vi "create_roi_file.vi"(7 "Data Files Path":path=path "C:/Users/QCC/Documents/Cesium_project/LabVIEW Projects/data/2011_03_02", 8 "error in (no error)":errorcluster, 9 "iteration string":string, 10 "date/time string":string, 11 "Camera in":refnum<class "Camera.lvclass">) -> (0 "error out":errorcluster, 3 "Camera out":refnum<class "Camera.lvclass">)   [LabVIEW 2013, in "Camera.lvclass"]
uses:
  Camera.lvclass
  Camera.lvclass/Camera.ctl
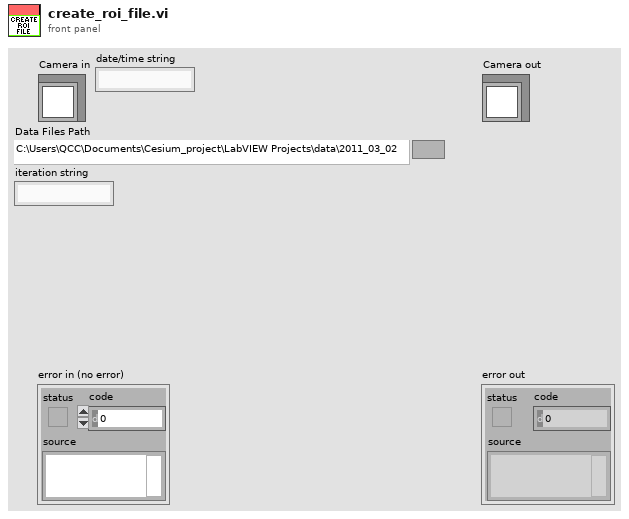
[diagram p1: front panel]
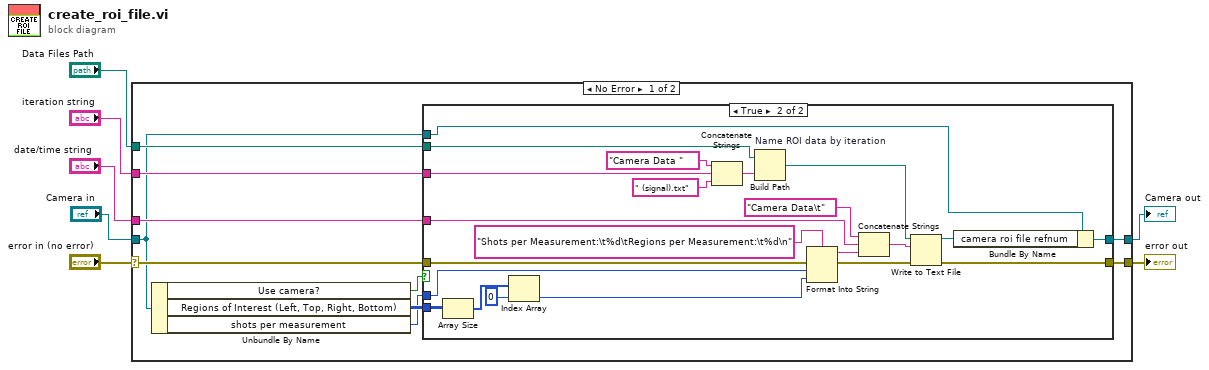
[diagram p0: block diagram]
diagram:
  n1 = case shown="No Error" "error in (no error)" {
    selector: "error in (no error)" -> [w15 w43]
    tunnel: [w14 w43] -> w6
    tunnel: [w8 w42] -> w4
    tunnel: "Camera in" -> [w9 w42]
    tunnel: "Data Files Path" -> [w17 _]
    tunnel: "date/time string" -> [w16 _]
    tunnel: "iteration string" -> [w13 _]
    frame No Error {
      n2 = Unbundle By Name(w9) -> ("Use camera?"=w12:bool, "Regions of Interest (Left, Top, Right, Bottom)"=w11:i32[][], "shots per measurement"=w10:i32)
      n3 = case shown="True" w12 {
        tunnel: w17 -> [_ w32]
        tunnel: w16 -> [_ w31]
        tunnel: w15 -> [w19 w28]
        tunnel: [w19 w30] -> w14
        tunnel: w13 -> [_ w29]
        tunnel: w11 -> [_ w27]
        tunnel: w10 -> [_ w24]
        tunnel: w9 -> [w18 w21]
        tunnel: [w18 w20] -> w8
        frame False {
        }
        frame True {
          n4 = Array Size(array=w27) -> (size(s)=w26:i32[])
          n5 = Index Array(array=w26, index=0) -> (element=w23:i32)
          n6 = Concatenate Strings("Camera Data ", w29, " (signal).txt" ("string")) -> (w40:string)
          n7 = Build Path "Name ROI data by iteration"(base path=w32, name or relative path=w40) -> (appended path=w41:path)
          n8 = Format Into String(format string="Shots per Measurement:\t%d\tRegions per Measurement:\t%d\n", error in=w28, w24, w23) -> (resulting string=w35:string, error out=w34:errorcluster)  [unwired: 1 in]
          n9 = Concatenate Strings("Camera Data\t", w31, w35) -> (w37:string)
          n10 = Write to Text File(file (use dialog)=w41, text=w37, error in=w34) -> (refnum out=w22:refnum<file>, error out=w30:errorcluster)  [unwired: 1 in, 1 out]
          n11 = Bundle By Name(cluster=w21, "camera roi file refnum"=w22) -> (w20:refnum<class "Camera.lvclass">)
        }
      }
    }
    frame Error {
    }
  }
  "error out" <- w6
  "Camera out" <- w4
